vi "PlayFile.vi"(11 "Old Files":T1[](array[typedef])) -> ()   [LabVIEW 2022 SP3]
uses:
  Curtin1_Label.ctl
panel:
  in  "Save Button":bool
  in  "Play Button":bool
  in  "Instruments":u16(ring) items=["JacksonStrad H.AvR"]
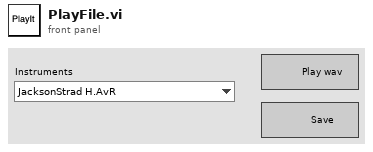
[diagram p1: front panel]
types:
  T1 = typedef "Curtin1_Label.ctl" = cluster{"Show?":bool, "Name":string, "Color":u32, "Path":path, "Show Notes":bool}
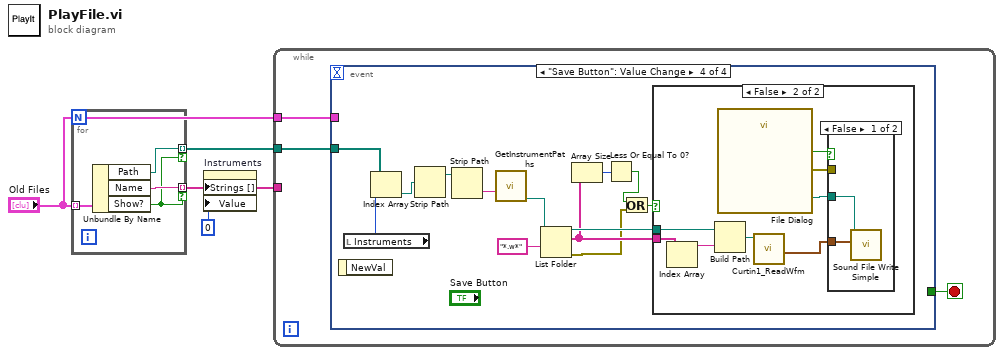
[diagram p0: block diagram]
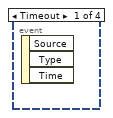
[diagram p2: hidden frame]
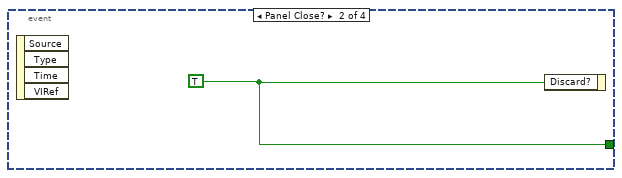
[diagram p3: hidden frame]
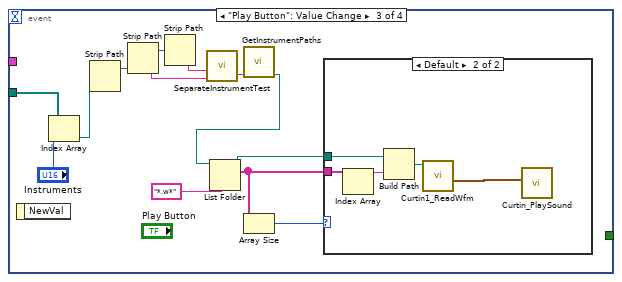
[diagram p4: hidden frame]
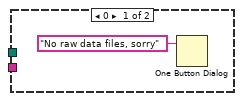
[diagram p5: hidden frame]
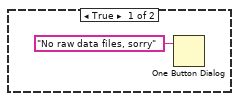
[diagram p6: hidden frame]
diagram:
  n1 = for {
    tunnel: "Old Files" -> [w8] mode=indexing
    tunnel: [w7] -> w3 mode=indexing if=w5
    tunnel: [w6] -> w2 mode=indexing if=w5
    n2 = Unbundle By Name(w8) -> ("Path"=w6:path, "Name"=w7:string, "Show?"=w5:bool)
  }
  n3 = property on="Instruments" class="Ring (strict)"("Strings []"=w3, "Value"=0) -> ()  [unwired: 2 in, 2 out]
  n4 = while {
    tunnel: w3 -> [_]
    tunnel: w2 -> [w10]
    tunnel: "Old Files" -> [w9]
    stop <- w11 stop-if-true
    n5 = event shown="[3] \"Save Button\": Value Change" {
      selector: _ -> [_ _ _ _]
      dyn-events: _ -> [_ _ _ _]
      timeout: _ -> [_ _ _ _]
      tunnel: [_ w12 _ _] -> w11
      tunnel: w10 -> [_ _ w21 w41]
      tunnel: w9 -> [_ _ _ _]
      event Timeout {
        n6 = event-data() -> ()  [unwired: 1 in, 3 out]
      }
      event Panel Close? {
        w12 = TRUE ("Discard?")
        n7 = event-data() -> ()  [unwired: 1 in, 4 out]
        n8 = event-data("Discard?"=w12) -> ()  [unwired: 1 in, 1 out]
      }
      event "Play Button": Value Change {
        n9 = event-data() -> ()  [unwired: 1 in, 1 out]
        n10 = Index Array(array=w21, index="Instruments") -> (element=w13:path)
        n11 = Strip Path(path=w13) -> (stripped path=w20:path)  [unwired: 1 out]
        n12 = Strip Path(path=w20) -> (stripped path=w19:path, name=w17:string)
        n13 = Strip Path(path=w19) -> (name=w18:string)  [unwired: 1 out]
        n14 = call "SeparateInstrumentTest.vi"("test in"=w17, "Instrument in"=w18) -> ("Instrument -- test out"=w16:string)  [unwired: 5 in, 4 out]
        n15 = call "GetInstrumentPaths.vi"("Instrument"=w16) -> ("Path To Raw Folder"=w24:path)  [unwired: 6 in, 4 out]
        n16 = List Folder(path=w24, pattern="*.w*") -> (path out=w22:path, filenames=w15:string[])  [unwired: 2 in, 2 out]
        n17 = Array Size(array=w15) -> (size(s)=w14:i32)
        n18 = case shown="Default" w14 {
          tunnel: w22 -> [_ w30]
          tunnel: w15 -> [_ w29]
          frame 0 {
            n19 = One Button Dialog(message="No raw data files, sorry") -> ()  [unwired: 1 in, 1 out]
          }
          frame Default {
            n20 = Index Array(array=w29) -> (element=w31:string)  [unwired: 1 in]
            n21 = Build Path(base path=w30, name or relative path=w31) -> (appended path=w28:path)
            n22 = call "Curtin1_ReadWfm.vi"("appended path"=w28) -> ("all waveforms in record"=w27:waveform(dbl)[])  [unwired: 9 in, 1 out]
            n23 = call "Curtin_PlaySound.vi"("all waveforms"=w27) -> ()  [unwired: 10 in, 1 out]
          }
        }
      }
      event "Save Button": Value Change {
        n24 = event-data() -> ()  [unwired: 1 in, 1 out]
        n25 = local read "Instruments"() -> (w37:u16)
        n26 = Index Array(array=w41, index=w37) -> (element=w39:path)
        n27 = Strip Path(path=w39) -> (stripped path=w38:path)  [unwired: 1 out]
        n28 = Strip Path(path=w38) -> (name=w40:string)  [unwired: 1 out]
        n29 = call "GetInstrumentPaths.vi"("Instrument"=w40) -> ("Path To Raw Folder"=w44:path)  [unwired: 6 in, 4 out]
        n30 = List Folder(path=w44, pattern="*.w*") -> (path out=w42:path, filenames=w36:string[], error out=w33:errorcluster)  [unwired: 2 in, 1 out]
        n31 = Array Size(array=w36) -> (size(s)=w35:i32)
        n32 = Less Or Equal To 0?(x=w35) -> (x <= 0?=w34:bool)
        n33 = Or(x=w34, y=w33) -> (x .or. y?=w32:bool)
        n34 = case shown="False" w32 {
          tunnel: w36 -> [_ w53]
          tunnel: w42 -> [_ w51]
          frame True {
            n35 = One Button Dialog(message="No raw data files, sorry") -> ()  [unwired: 1 in, 1 out]
          }
          frame False {
            n36 = Index Array(array=w53) -> (element=w52:string)  [unwired: 1 in]
            n37 = Build Path(base path=w51, name or relative path=w52) -> (appended path=w50:path)
            n38 = call "File Dialog"() -> ("selected path"=w48:path, "cancelled"=w47:bool, "error out"=w46:errorcluster)  [unwired: 12 in, 1 out]
            n39 = call "Curtin1_ReadWfm.vi"("appended path"=w50) -> ("all waveforms in record"=w49:waveform(dbl)[])  [unwired: 9 in, 1 out]
            n40 = case shown="False" w47 {
              tunnel: w49 -> [w55 _]
              tunnel: w48 -> [w54 _]
              tunnel: w46 -> [_ _]
              frame False {
                n41 = call <vilib>:"Sound File Write Simple.vi"("data"=w55, "path"=w54) -> ()  [unwired: 8 in, 2 out]
              }
              frame True {
              }
            }
          }
        }
      }
    }
  }
